vi "Reserve Session.vi"(6 "timeout in milliseconds":i32, 8 "error in":errorcluster, 9 "instrument type ID":string, 10 "pin or relay names":string[](array[string]), 11 "Measurement Context In":refnum<class "MeasurementContext.lvclass">) -> (0 "error out":errorcluster, 1 "gRPC device location":T3, 2 "session information":T4, 3 "Measurement Context out":refnum<class "MeasurementContext.lvclass">, 5 "gRPC channel pool out":T1)   [LabVIEW 2020]
uses:
  <vilib>/MeasurementLink/MeasurementLink Session Management Client/RPC Messages/ni_measurementlink_sessionmanagement_v1_SessionInformation.ctl
  <vilib>/MeasurementLink/MeasurementLink Session Management Client/RPC Messages/nidevice_grpc_Session.ctl
  <vilib>/MeasurementLink/MeasurementLink Session Management Client/RPC Messages/ni_measurementlink_sessionmanagement_v1_ChannelMapping.ctl
  <vilib>/MeasurementLink/MeasurementLink Discovery Client/RPC Messages/ni_measurementlink_discovery_v1_ServiceLocation.ctl
  GRPC Channel Pool.ctl
  <vilib>/gRPC/LabVIEW gRPC Library/Shared/grpcId.ctl
  <vilib>/MeasurementLink/MeasurementLink Measurement Server/Classes/MeasurementContext/MeasurementContext.lvclass
  NIDCPowerSourceDCVoltage.lvlib
  <vilib>/MeasurementLink/MeasurementLink Session Management Client/MeasurementLink Session Management Client.lvlib
  <vilib>/MeasurementLink/MeasurementLink Discovery Client/MeasurementLink Discovery Client.lvlib
  <vilib>/gRPC/LabVIEW gRPC Library/grpc-lvsupport-release.lvlib
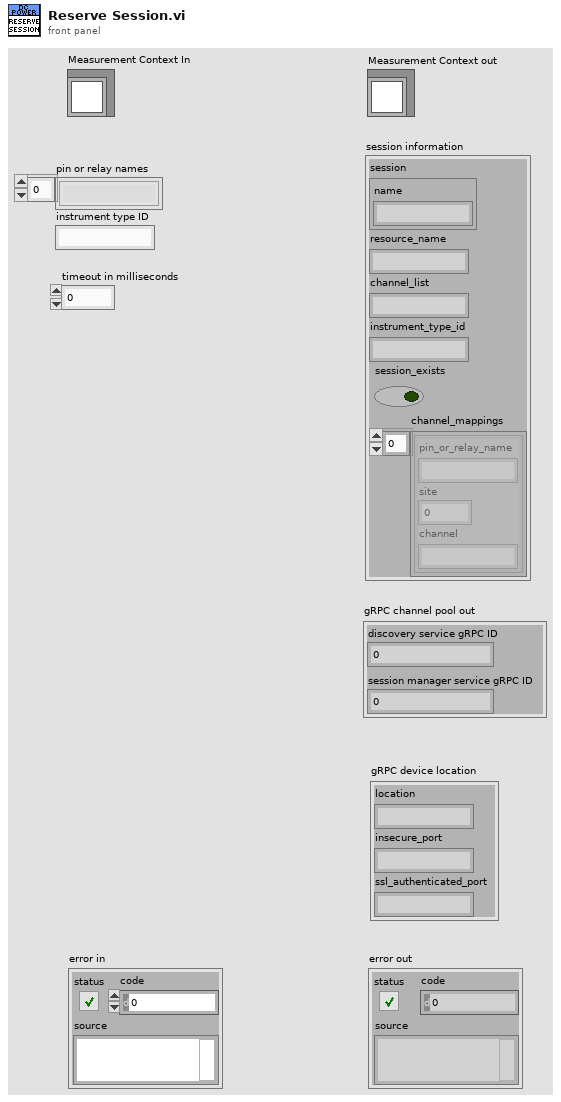
[diagram p1: front panel]
types:
  T1 = typedef "NIDCPowerSourceDCVoltage.lvlib/GRPC Channel Pool.ctl" = cluster{"discovery service gRPC ID":T2, "session manager service gRPC ID":T2}
  T2 = typedef "grpc-lvsupport-release.lvlib/grpcId.ctl" = u64
  T3 = typedef "MeasurementLink Discovery Client.lvlib/ni_measurementlink_discovery_v1_ServiceLocation.ctl" = cluster{"location":string, "insecure_port":string, "ssl_authenticated_port":string}
  T4 = typedef "MeasurementLink Session Management Client.lvlib/ni_measurementlink_sessionmanagement_v1_SessionInformation.ctl" = cluster{"session":T5, "resource_name":string, "channel_list":string, "instrument_type_id":string, "session_exists":bool, "channel_mappings":T6[]}
  T5 = typedef "MeasurementLink Session Management Client.lvlib/nidevice_grpc_Session.ctl" = cluster{"name":string}
  T6 = typedef "MeasurementLink Session Management Client.lvlib/ni_measurementlink_sessionmanagement_v1_ChannelMapping.ctl" = cluster{"pin_or_relay_name":string, "site":i32, "channel":string}
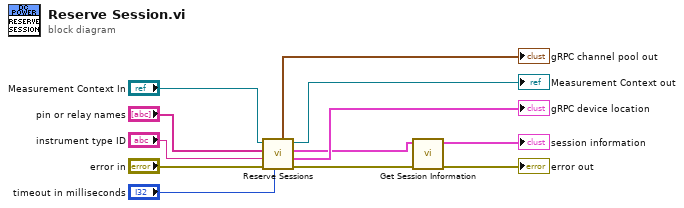
[diagram p0: block diagram]
diagram:
  n1 = call "Reserve Sessions.vi"("timeout in milliseconds"="timeout in milliseconds", "error in"="error in", "instrument type ID"="instrument type ID", "pin or relay names"="pin or relay names", "Measurement Context In"="Measurement Context In") -> ("error out"=w9:errorcluster, "gRPC device location"=→"gRPC device location":T3, "session information"=w1:T4[], "Measurement Context out"=→"Measurement Context out":refnum<class "MeasurementContext.lvclass">, "gRPC channel pool out"=→"gRPC channel pool out":T1)  [unwired: 2 in]
  n2 = call "Get Session Information.vi"("error in (no error)"=w9, "session information"=w1) -> ("error out"=→"error out":errorcluster, "session information"=→"session information":T4)  [unwired: 8 in]
